vi "CallRunOperation.vi"(7 "Logger":refnum<class "Logger.lvclass">, 8 "Inputs":string[](array[string]), 9 "CoreOperation in":refnum<class "CoreOperation.lvclass">) -> (1 "Output/Failure":string, 2 "CLI Process Return Code":i32, 3 "CoreOperation out":refnum<class "CoreOperation.lvclass">)   [LabVIEW 2014, in "CoreOperation.lvclass"]
uses:
  CoreOperation.lvclass
  Utilities/Logger/Logger.lvclass
  CoreOperation.lvclass/CoreOperation.ctl
panel:
  in  "Empty help message":string="This operation has no documentation defined"
  in  "Usage":string="Usage: "
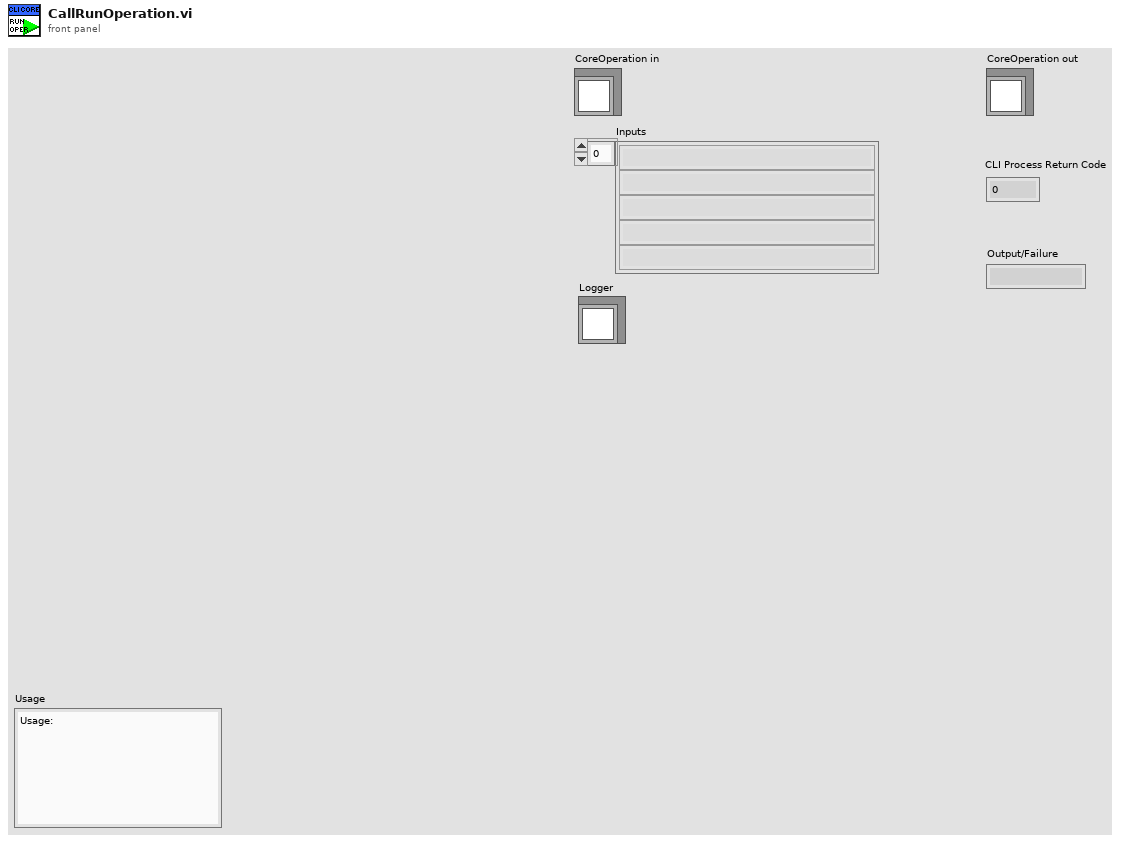
[diagram p1: front panel]
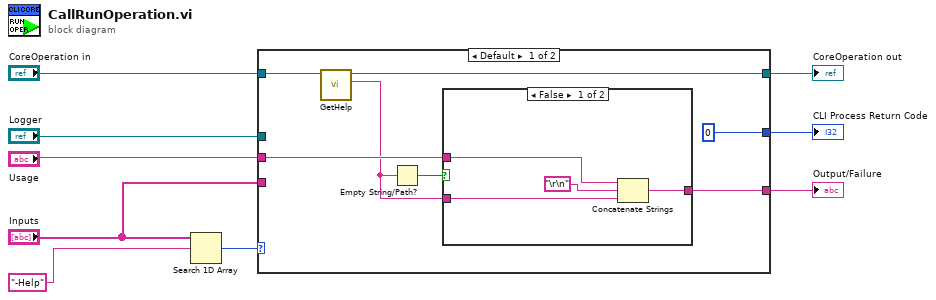
[diagram p0: block diagram]
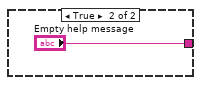
[diagram p2: hidden frame]
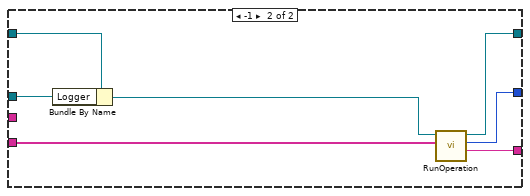
[diagram p3: hidden frame]
diagram:
  n1 = Search 1D Array(1D array="Inputs", element="-Help" ("\"-help\" string")) -> (index of element=w1:i32)  [unwired: 1 in]
  n2 = case shown="Default" w1 {
    tunnel: [w15 w28] -> w7
    tunnel: "Inputs" -> [_ w23]
    tunnel: "CoreOperation in" -> [w16 w27]
    tunnel: "Logger" -> [_ w25]
    tunnel: [0 ("CLI Process Return Code") w22] -> w5
    tunnel: [w12 w24] -> w4
    tunnel: "Usage" -> [w11 _]
    frame Default {
      n3 = call-dynamic "GetHelp.vi"("CoreOperation in"=w16) -> ("Help"=w10:string, "CoreOperation out"=w15:refnum<class "CoreOperation.lvclass">)  [unwired: 9 in]
      n4 = Empty String/Path?(string/path=w10) -> (empty?=w13:bool)
      n5 = case shown="False" w13 {
        tunnel: [w17 "Empty help message"] -> w12
        tunnel: w11 -> [w19 _]
        tunnel: w10 -> [w18 _]
        frame False {
          n6 = Concatenate Strings(w19, "\r\n", w18) -> (w17:string)
        }
        frame True {
        }
      }
    }
    frame -1 {
      n7 = Bundle By Name(cluster=w27, "Logger"=w25) -> (w26:refnum<class "CoreOperation.lvclass">)
      n8 = call-dynamic "RunOperation.vi"("Inputs"=w23, "CoreOperation in"=w26) -> ("Output/Failure"=w24:string, "CLI Process Return Code"=w22:i32, "CoreOperation out"=w28:refnum<class "CoreOperation.lvclass">)  [unwired: 7 in]
    }
  }
  "CoreOperation out" <- w7
  "CLI Process Return Code" <- w5
  "Output/Failure" <- w4
